vi "Dijkstras algorithm.vi"(11 "Map":u8[][](array[numeric])) -> (3 "Array":i32[][](array[numeric]))   [LabVIEW 2020, in "2021_15.lvclass"]
uses:
  2021_15.lvclass
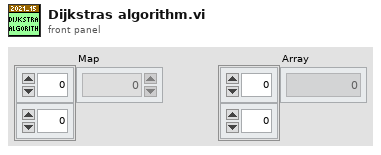
[diagram p1: front panel]
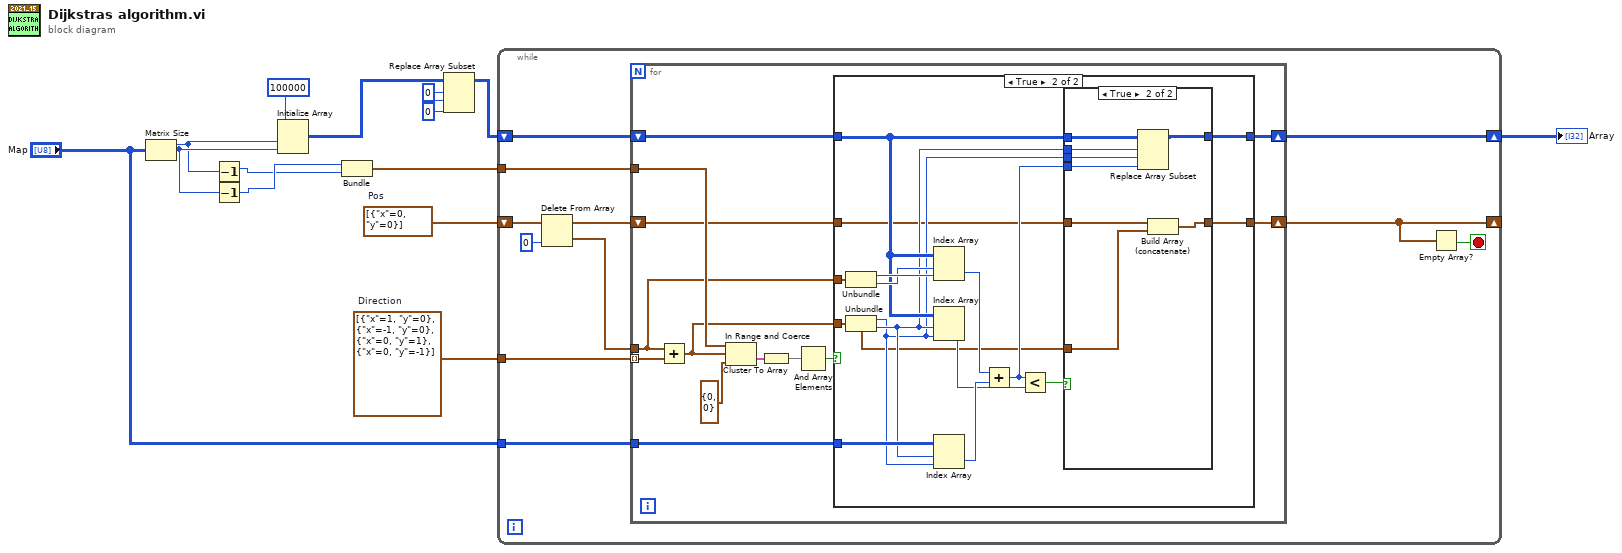
[diagram p0: block diagram]
diagram:
  w6 = 0 ("index (row)")
  w2 = cluster{"x":i32, "y":i32}[] [{"x"=1, "y"=0}, {"x"=-1, "y"=0}, {"x"=0, "y"=1}, {"x"=0, "y"=-1}]  # Direction
  w1 = cluster{"x":i32, "y":i32}[] [{"x"=0, "y"=0}]  # Pos
  n1 = Matrix Size(0:"Map") -> (1:w3:i32, 2:w4:i32)
  n2 = Decrement(x=w3) -> (x-1=w11:i32)
  n3 = Decrement(x=w4) -> (x-1=w12:i32)
  n4 = Initialize Array(100000 ("element"), w3, w4) -> (w8:i32[][])
  n5 = Bundle(w12, w11) -> (w5:cluster{i32, i32})  [unwired: 1 in]
  n6 = Replace Array Subset(array=w8, new element=0 ("new element/subarray"), index (row)=w6, index (col)=w6) -> (w9:i32[][])
  n7 = while {
    shift-right: [w15] -> _
    shift-left: w1 -> [w24]
    tunnel: w2 -> [w21]
    shift-right: [w17] -> w10
    shift-left: w9 -> [w20]
    tunnel: w5 -> [w19]
    tunnel: "Map" -> [w18]
    stop <- w25 stop-if-true
    n8 = Delete From Array(array=w24, index=0) -> (deleted portion=w22:cluster{"x":i32, "y":i32}, array with subset deleted=w16:cluster{"x":i32, "y":i32}[])  [unwired: 1 in]
    n9 = for {
      tunnel: w22 -> [w29]
      tunnel: w21 -> [w38] mode=indexing
      shift-right: [w28] -> w17
      shift-left: w20 -> [w31]
      tunnel: w19 -> [w36]
      tunnel: w18 -> [w30]
      shift-right: [w26] -> w15
      shift-left: w16 -> [w27]
      n10 = Add(x=w29, y=w38) -> (x+y=w32:cluster{"x":i32, "y":i32})
      n11 = In Range and Coerce(upper limit=w36, x=w32, lower limit=cluster{"x":i32, "y":i32} {"x"=0, "y"=0}) -> (In Range?=w35:cluster{"x":bool, "y":bool})  [unwired: 1 out]
      n12 = Cluster To Array(cluster=w35) -> (array=w34:bool[])
      n13 = And Array Elements(Boolean array=w34) -> (logical AND=w33:bool)
      n14 = case shown="True" w33 {
        tunnel: w32 -> [_ w41]
        tunnel: w31 -> [w40 w48]
        tunnel: w30 -> [_ w56]
        tunnel: w29 -> [_ w54]
        tunnel: [w40 w47] -> w28
        tunnel: w27 -> [w39 w43]
        tunnel: [w39 w42] -> w26
        frame False {
        }
        frame True {
          n15 = Unbundle(w54) -> ("x"=w53:i32, "y"=w52:i32)
          n16 = Unbundle(w41) -> ("x"=w45:i32, "y"=w46:i32)
          n17 = Index Array(array=w48, index (row)=w52, index (col)=w53) -> (element=w51:i32)
          n18 = Index Array(array=w48, index (row)=w46, index (col)=w45) -> (element=w50:i32)
          n19 = Index Array(array=w56, index (row)=w46, index (col)=w45) -> (element=w55:u8)
          n20 = Add(x=w51, y=w55) -> (x+y=w44:i32)
          n21 = Less?(x=w44, y=w50) -> (x < y?=w49:bool)
          n22 = case shown="True" w49 {
            tunnel: w48 -> [w58 w66]
            tunnel: [w58 w65] -> w47
            tunnel: w46 -> [_ w64]
            tunnel: w45 -> [_ w63]
            tunnel: w44 -> [_ w62]
            tunnel: w43 -> [w57 w61]
            tunnel: [w57 w60] -> w42
            tunnel: w41 -> [_ w59]
            frame False {
            }
            frame True {
              n23 = Replace Array Subset(array=w66, new element=w62, index (row)=w64, index (col)=w63) -> (w65:i32[][])
              n24 = Build Array (concatenate)(w61, w59) -> (w60:cluster{"x":i32, "y":i32}[])
            }
          }
        }
      }
    }
    n25 = Empty Array?(array=w15) -> (empty?=w25:bool)
  }
  "Array" <- w10
